vi "Apply ROI mask.vi"(9 "ROI":T1, 11 "Refnum in":T2) -> (3 "Masked":T2(plugin-control))   [LabVIEW 2013]
uses:
  <vilib>/vision/Image Controls.llb/IMAQ Image.ctl
  <vilib>/vision/NI_Vision_Development_Module.lvlib
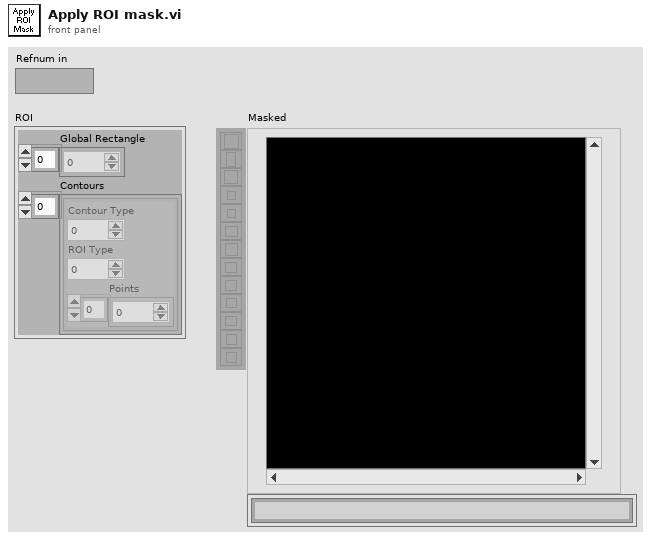
[diagram p1: front panel]
types:
  T1 = cluster{"Global Rectangle":i32[], "Contours":cluster{"Contour Type":u32, "ROI Type":u32, "Points":i32[]}[]}
  T2 = typedef "IMAQ Image.ctl" = refnum<image>
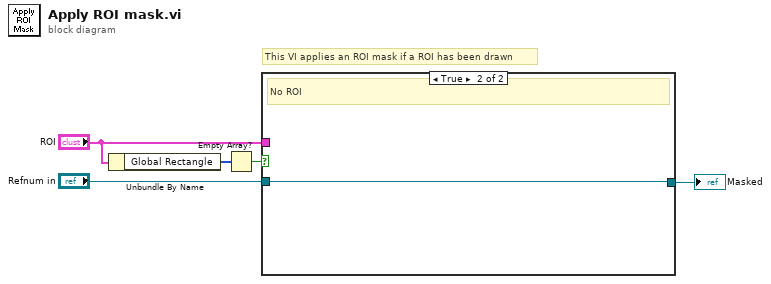
[diagram p0: block diagram]
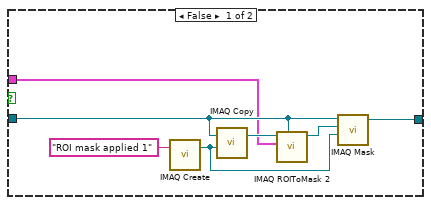
[diagram p2: hidden frame]
diagram:
  # "This VI applies an ROI mask if a ROI has been drawn"
  n1 = Unbundle By Name("ROI") -> ("Global Rectangle"=w2:i32[])
  n2 = Empty Array?(array=w2) -> (empty?=w1:bool)
  n3 = case shown="True" w1 {
    tunnel: [w12 w13] -> w5
    tunnel: "Refnum in" -> [w9 w13]
    tunnel: "ROI" -> [w6 _]
    frame False {
      n4 = call "IMAQ Create"("Image Name"="ROI mask applied 1") -> ("New Image"=w11:T2)  [unwired: 4 in, 1 out]
      n5 = call "IMAQ Copy"("Image Dst"=w11, "Image Src"=w9) -> ("Image Dst Out"=w8:T2)  [unwired: 4 in, 1 out]
      n6 = call "IMAQ ROIToMask 2"("Image Model"=w9, "ROI Descriptor"=w6, "Image"=w8) -> ("Image Out"=w10:T2)  [unwired: 6 in, 2 out]
      n7 = call "IMAQ Mask"("Image Dst"=w11, "Image Mask"=w10, "Image Src"=w9) -> ("Image Dst Out"=w12:T2)  [unwired: 2 in, 1 out]
    }
    frame True {
      # "No ROI"
    }
  }
  "Masked" <- w5
